vi "SetExpAuto.vi"   [LabVIEW 2012]
uses:
  <vilib>/Rock Robotics/WPI/Relay/WPI_RelayValue.ctl
  <vilib>/Rock Robotics/WPI/Camera/WPI_CameraExposure Values.ctl
panel:
  # "This vi sets exposure for vision processing"
types:
  T1 = typedef "WPI_ServoDeviceRef.ctl" = cluster{"DeviceStatus":errorcluster, "Digital Module":T2, "PWM Channel":T3, "DeadBand":T4}
  T2 = typedef "FPGA_TypedefDigitalModule.ctl" = enum16{"Digital Module 1", "Digital Module 2"}
  T3 = typedef "FPGA_DIOPWMChannel.ctl" = enum8{"PWM 1", "PWM 2", "PWM 3", "PWM 4", "PWM 5", "PWM 6", "PWM 7", "PWM 8", "PWM 9", "PWM 10", "Invalid"}
  T4 = typedef "WPI_PWMDeadband.ctl" = cluster{"Name":string, "maxPositivePwm":i32, "minPositivePwm":i32, "centerPwm":i32, "maxNegativePwm":i32, "minNegativePwm":i32, "angularRange":u16}
  T5 = typedef "WPI_CameraDevRef.ctl" = cluster{"Camera Address":string, "CameraStatus":errorcluster, "Acquire Image Notifier":refnum<notifier>}
  T6 = typedef "WPI_RelayDevRef.ctl" = cluster{"DevStatus":errorcluster, "Relay Channel":T7, "Digital Module":T2, "Relay Direction":T8}
  T7 = typedef "FPGA_DIORelayChannel.ctl" = enum8{"Relay 1", "Relay 2", "Relay 3", "Relay 4", "Relay 5", "Relay 6", "Relay 7", "Relay 8", "Invalid"}
  T8 = typedef "WPI_RelayDirection.ctl" = enum16{"Both directions", "Forward only", "Reverse only"}
  T9 = typedef "WPI_RelayValue.ctl" = enum16{"Off", "On", "Forward", "Reverse"}
  T10 = typedef "WPI_CameraExposure Values.ctl" = enum16{"Auto", "Flicker-free 50 Hz", "Flicker-free 60 Hz", "Hold current"}
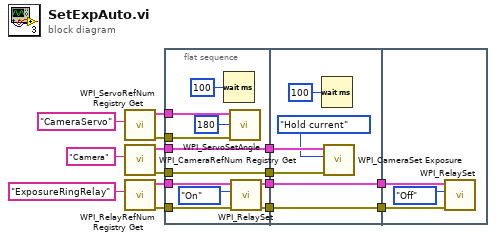
[diagram p0: block diagram]
diagram:
  n1 = call <vilib>:"WPI_ServoRefNum Registry Get.vi"("refnum name"="CameraServo") -> ("error out"=w8:errorcluster, "ServoDeviceRef"=w9:T1)  [unwired: 9 in]
  n2 = call <vilib>:"WPI_CameraRefNum Registry Get.vi"("refnum name"="Camera") -> ("error out"=w13:errorcluster, "CameraDevRef"=w11:T5)  [unwired: 9 in]
  n3 = call <vilib>:"WPI_RelayRefNum Registry Get.vi"("refnum name"="ExposureRingRelay") -> ("error out"=w14:errorcluster, "RelayDevRef"=w15:T6)  [unwired: 9 in]
  n4 = flat-sequence {
    tunnel: w15 -> [w25]
    tunnel: w14 -> [w24]
    tunnel: w13 -> [w23]
    tunnel: [w23] -> w12
    tunnel: w11 -> [w22]
    tunnel: [w22] -> w10
    tunnel: w9 -> [w21]
    tunnel: w8 -> [w20]
    tunnel: [w19] -> w6
    tunnel: [w18] -> w4
    tunnel: w12 -> [w32]
    tunnel: w10 -> [w31]
    tunnel: [w29] -> w7
    tunnel: w6 -> [w29]
    tunnel: [w28] -> w5
    tunnel: w4 -> [w28]
    tunnel: w7 -> [w35]
    tunnel: w5 -> [w34]
    frame #0 {
      n5 = Wait (ms)(milliseconds to wait=u32 100) -> ()  [unwired: 1 out]
      n6 = call <vilib>:"WPI_ServoSetAngle.vi"("error in (no error)"=w20, "Angle"=180, "ServoDeviceRef"=w21) -> ()  [unwired: 7 in, 2 out]
      n7 = call <vilib>:"WPI_RelaySet.vi"("error in (no error)"=w24, "RelayValue"=WPI_RelayValue."On", "RelayDevRef"=w25) -> ("error out"=w18:errorcluster, "RelayDevRef"=w19:T6)  [unwired: 7 in]
    }
    frame #1 {
      n8 = Wait (ms)(milliseconds to wait=u32 100) -> ()  [unwired: 1 out]
      n9 = call <vilib>:"WPI_CameraSet Exposure.vi"("error in (no error)"=w32, "Exposure"=WPI_CameraExposure_Values."Hold current", "CameraDevRef"=w31) -> ()  [unwired: 7 in, 2 out]
    }
    frame #2 {
      n10 = call <vilib>:"WPI_RelaySet.vi"("error in (no error)"=w34, "RelayValue"=WPI_RelayValue."Off", "RelayDevRef"=w35) -> ()  [unwired: 7 in, 2 out]
    }
  }
